vi "N-Double FFT Mesurament (Control - Init Wave&Window - Snapshot - DoubleFFT - Latency - Low Freq) RT Test.vi"() -> ()   [LabVIEW 2014]
uses:
  <vilib>/FPGAPlugInAG/sbRIO-9636/niLvFpga_Open_sbRIO-9636.vi
  <vilib>/rvi/interface/common/dynamic/niFpgaDynamicAddResources.vi
  <vilib>/Utility/error.llb/Error Cluster From Error Code.vi
  <vilib>/rvi/errors/niLvFpgaAdjustHostInterfaceError.vi
  <vilib>/rvi/interface/common/niFpgaWaitOnOcc.vi
  <vilib>/FPGAPlugInAG/Dynamic/niLvFpga_Run_Dynamic.vi
  <vilib>/FPGAPlugInAG/Dynamic/niLvFpga_Abort_Dynamic.vi
  <vilib>/FPGAPlugInAG/Dynamic/niLvFpga_Reset_Dynamic.vi
  <vilib>/FPGAPlugInAG/Dynamic/niLvFpga_Close_Dynamic.vi
  <vilib>/rvi/interface/nirviOpenFPGA/nirviOpenFPGA.xnode
  FPGA Bitfiles/LaserDistanceSen_FPGATarget_DoubleFFTMesuram_rbFcbbMisXs.lvbitx
  FPGA Target/Test VIs/Double FFT Mesurament (Control - Init Wave&Window - Snapshot - DoubleFFT - Latency - Low Freq - PARAM LEO) test.vi
  <vilib>/rvi/interface/nirviReadWriteControl/nirviReadWriteControl.xnode
  <vilib>/rvi/interface/nirviMethod/nirviMethod.xnode
  <vilib>/rvi/interface/nirviCloseFPGA/nirviCloseFPGA.xnode
  <vilib>/FPGAPlugInAG/Dynamic/niLvFpga_ConfigureFifo_Dynamic.vi
  <vilib>/rvi/errors/niLvFpgaMergeErrorWithErrorCode.vi
  <vilib>/FPGAPlugInAG/Dynamic/niLvFpga_StartFifo_Dynamic.vi
  <vilib>/rvi/interface/Simulation/niFpgaSimulationCallBeginRW.vi
  <vilib>/FPGAPlugInAG/Dynamic/niLvFpga_ReadFifo_Dynamic.vi
  NiFpgaLv.dll
panel:
  out "error out":errorcluster
  out "N-FFT":dbl[](graph)
  out "Write memory complete":bool
  in  "#Signals":u32=1
  in  "stop":bool
  in  "Initial Latency points":u32(slide)=10 scale=0.0..1249.0
  out "Elements Remaining FFT":u32
  out "Elements Remaining Signal":u32
  out "N-Signals":dbl[](graph)
  in  "Snapshot":bool
  in  "Windowing":T1(ring)
  in  "first bin":i32=15
  in  "last bin":i32=255
  in  "lower limit 2":u32(slide)=725 scale=625.0..738.0
  in  "lower limit 1":u32(slide)=100 scale=0.0..113.0
  # "WARNING:\nOnce pressed wait untill the end of operation"
  # "OFFLINE parameters"
  # "Max Detection FFT bin range"
  # "TEST"
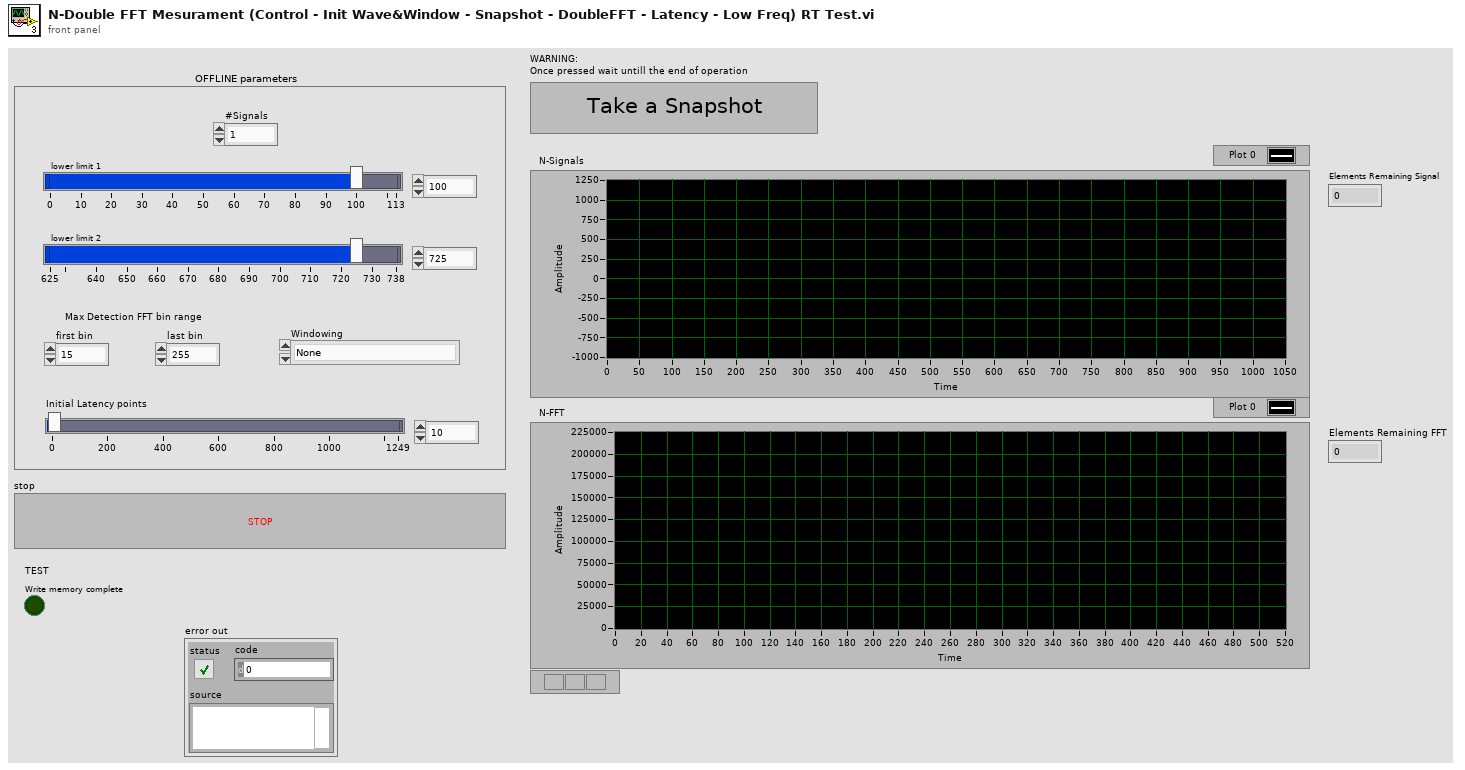
[diagram p1: front panel]
types:
  T1 = enum16{"None", "Hanning", "Hamming", "Blackman", "Blackman-Harris"}
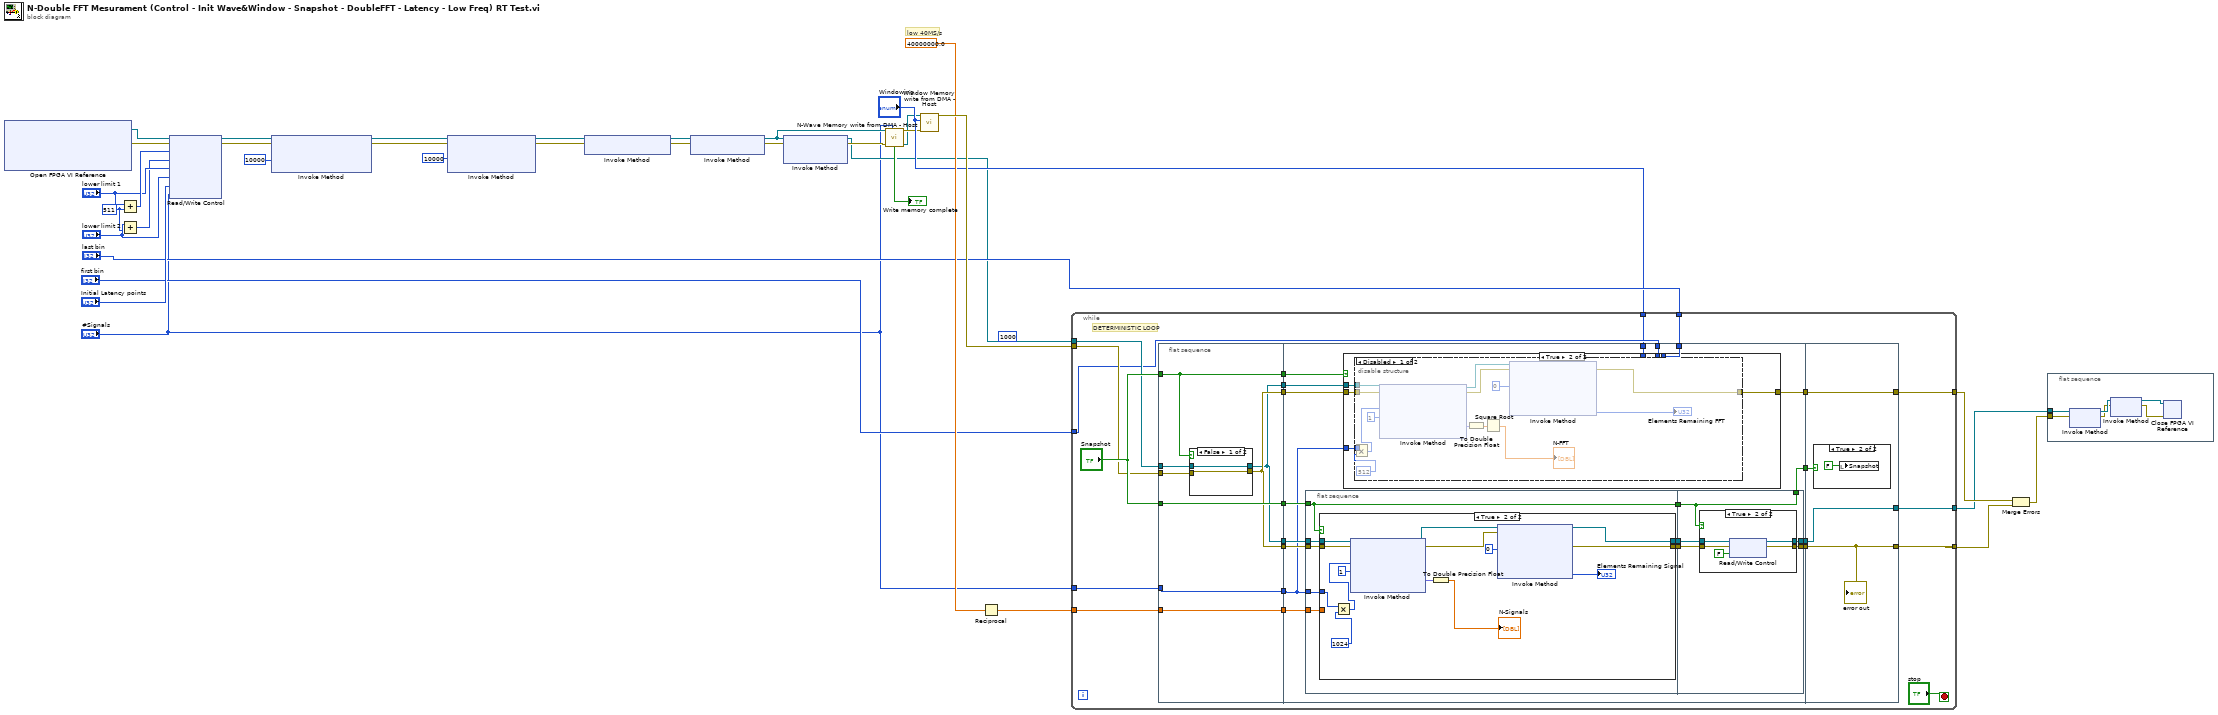
[diagram p0: block diagram]
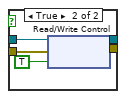
[diagram p2: hidden frame]
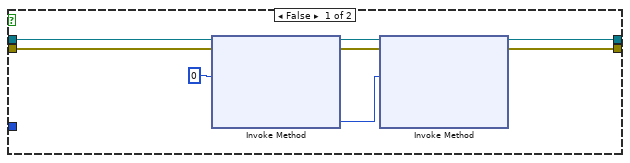
[diagram p3: hidden frame]
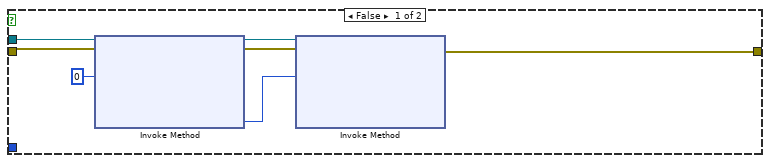
[diagram p5: hidden frame]
diagram:
  (unwired) i64 1000 ("Period")
  w32 = u32 511 ("y")
  # "low 40MS/s"
  n1 = xnode "Open FPGA VI Reference"() -> ("FPGA VI Reference Out"=w31:refnum<k20>, "error out"=w30:errorcluster)  [unwired: 2 in]
  n2 = Add(x="lower limit 1", y=w32) -> (x+y=w36:u32)
  n3 = Add(x="lower limit 2", y=w32) -> (x+y=w34:u32)
  n4 = xnode "Read/Write Control"("FPGA VI Reference In"=w31, "error in"=w30, "upper limit 1"=w36, "upper limit 2"=w34, "lower limit 1"="lower limit 1", "lower limit 2"="lower limit 2", "Latency points"="Initial Latency points", "n"="#Signals") -> ("FPGA VI Reference Out"=w28:refnum<k20>, "error out"=w27:errorcluster)
  n5 = xnode "Invoke Method"("FPGA VI Reference In"=w28, "error in"=w27, "Requested Depth"=u32 10000) -> ("FPGA VI Reference Out"=w11:refnum<k20>, "error out"=w12:errorcluster)  [unwired: 1 out]
  n6 = xnode "Invoke Method"("FPGA VI Reference In"=w11, "error in"=w12, "Requested Depth"=u32 10000) -> ("FPGA VI Reference Out"=w20:refnum<k20>, "error out"=w21:errorcluster)  [unwired: 1 out]
  n7 = xnode "Invoke Method"("FPGA VI Reference In"=w20, "error in"=w21) -> ("FPGA VI Reference Out"=w9:refnum<k20>, "error out"=w10:errorcluster)
  n8 = xnode "Invoke Method"("FPGA VI Reference In"=w9, "error in"=w10) -> ("FPGA VI Reference Out"=w2:refnum<k20>, "error out"=w19:errorcluster)
  n9 = xnode "Invoke Method"("FPGA VI Reference In"=w2, "error in"=w19) -> ("FPGA VI Reference Out"=w3:refnum<k20>, "error out"=w7:errorcluster)  [unwired: 1 in]
  n10 = call "N-Wave Memory write from DMA - Host.vi"("n"="#Signals", "error in"=w7, "FPGA VI Reference In"=w2) -> ("FPGA VI Reference Out"=w5:refnum<k20>, "error out"=w6:errorcluster, "Write memory complete"=→"Write memory complete":bool)  [unwired: 6 in]
  n11 = call "Window Memory write from DMA - Host.vi"("error in"=w6, "Enum"="Windowing", "FPGA VI Reference In"=w5) -> ("error out"=w29:errorcluster)  [unwired: 5 in, 3 out]
  n12 = Reciprocal(x=40000000.0 ("Sample Rate (S/s)")) -> (1/x=w23:dbl)
  n13 = while {
    tunnel: w3 -> [w55]
    tunnel: w29 -> [w56]
    tunnel: [w58] -> w18
    tunnel: w23 -> [w60]
    tunnel: [w59] -> w17
    tunnel: "first bin" -> [w44]
    tunnel: "last bin" -> [w43]
    tunnel: [w41] -> w13
    tunnel: "Windowing" -> [w39]
    tunnel: "#Signals" -> [w37]
    stop <- "stop" stop-if-true
    # "DETERMINISTIC LOOP"
    n14 = flat-sequence {
      tunnel: w55 -> [w64]
      tunnel: w56 -> [w65]
      tunnel: "Snapshot" -> [w62]
      tunnel: "Snapshot" -> [w67]
      tunnel: w60 -> [w68]
      tunnel: [w66] -> w54
      tunnel: [w68] -> w53
      tunnel: [w67] -> w52
      tunnel: [w62] -> w51
      tunnel: [w66] -> w50
      tunnel: [w63] -> w49
      tunnel: [w63] -> w48
      tunnel: [w61] -> w38
      tunnel: w37 -> [w61]
      tunnel: w54 -> [w89]
      tunnel: w53 -> [w88]
      tunnel: w52 -> [w82]
      tunnel: w51 -> [w85]
      tunnel: w50 -> [w84]
      tunnel: w49 -> [w83]
      tunnel: w48 -> [w90]
      tunnel: [w87] -> w47
      tunnel: [w86] -> w46
      tunnel: [w81] -> w45
      tunnel: w44 -> [w80]
      tunnel: w43 -> [w79]
      tunnel: [w78] -> w40
      tunnel: w39 -> [w77]
      tunnel: w38 -> [w76]
      tunnel: [w162] -> w58
      tunnel: [w163] -> w59
      tunnel: w47 -> [w163]
      tunnel: w46 -> [w162]
      tunnel: w45 -> [w161]
      tunnel: [w160] -> w41
      tunnel: w40 -> [w160]
      frame #0 {
        n15 = case shown="False" w62 {
          tunnel: [w69 w74] -> w66
          tunnel: w65 -> [w69 w73]
          tunnel: w64 -> [w70 w72]
          tunnel: [w70 w71] -> w63
          frame False {
          }
          frame True {
            n16 = xnode "Read/Write Control"("FPGA VI Reference In"=w72, "error in"=w73, "snapshot"=TRUE) -> ("FPGA VI Reference Out"=w71:refnum<k20>, "error out"=w74:errorcluster)
          }
        }
      }
      frame #1 {
        n17 = flat-sequence {
          tunnel: w90 -> [w100]
          tunnel: w89 -> [w99]
          tunnel: w88 -> [w98]
          tunnel: w82 -> [w95]
          tunnel: [w97] -> w93
          tunnel: [w96] -> w92
          tunnel: [w95] -> w91
          tunnel: w76 -> [w94]
          tunnel: [w125] -> w86
          tunnel: w93 -> [w127]
          tunnel: w92 -> [w126]
          tunnel: w91 -> [w124]
          tunnel: [w124] -> w81
          tunnel: [w123] -> w78
          frame #0 {
            n18 = case shown="True" w95 {
              tunnel: w100 -> [w107 w122]
              tunnel: w99 -> [w105 w121]
              tunnel: [w104 w116] -> w96
              tunnel: w98 -> [_ _]
              tunnel: [w101 w115] -> w97
              tunnel: w94 -> [_ w112]
              frame False {
                n19 = xnode "Invoke Method"("FPGA VI Reference In"=w107, "error in"=w105, "Number of Elements"=u32 0) -> ("FPGA VI Reference Out"=w103:refnum<k20>, "error out"=w102:errorcluster, "Elements Remaining"=w106:u32)  [unwired: 1 in, 1 out]
                n20 = xnode "Invoke Method"("FPGA VI Reference In"=w103, "error in"=w102, "Number of Elements"=w106) -> ("FPGA VI Reference Out"=w101:refnum<k20>, "error out"=w104:errorcluster)  [unwired: 1 in, 2 out]
              }
              frame True {
                n21 = Multiply(x=w112, y=u32 1024 ("Number of Elements")) -> (x*y=w113:u32)
                n22 = xnode "Invoke Method"("FPGA VI Reference In"=w122, "error in"=w121, "Number of Elements"=w113, "Timeout (ms)"=1) -> ("FPGA VI Reference Out"=w118:refnum<k20>, "error out"=w117:errorcluster, "Data"=w120:fxp<+/-,12,12>[])  [unwired: 1 out]
                n23 = To Double Precision Float(number=w120) -> (double precision float=→"N-Signals":dbl[])
                n24 = xnode "Invoke Method"("FPGA VI Reference In"=w118, "error in"=w117, "Number of Elements"=u32 0) -> ("FPGA VI Reference Out"=w115:refnum<k20>, "error out"=w116:errorcluster, "Elements Remaining"=→"Elements Remaining Signal":u32)  [unwired: 1 in, 1 out]
              }
            }
          }
          frame #1 {
            n25 = case shown="True" w124 {
              tunnel: [w129 w132] -> w125
              tunnel: w127 -> [w128 w133]
              tunnel: w126 -> [w129 w131]
              tunnel: [w128 w130] -> w123
              frame False {
              }
              frame True {
                n26 = xnode "Read/Write Control"("FPGA VI Reference In"=w133, "error in"=w131, "snapshot"=FALSE) -> ("FPGA VI Reference Out"=w130:refnum<k20>, "error out"=w132:errorcluster)
              }
            }
          }
        }
        n27 = case shown="True" w85 {
          tunnel: w83 -> [w140 w144]
          tunnel: w84 -> [w137 w145]
          tunnel: [w136 w143] -> w87
          tunnel: w80 -> [_ _]
          tunnel: w79 -> [_ _]
          tunnel: w77 -> [_ _]
          tunnel: w76 -> [_ w142]
          frame False {
            n28 = xnode "Invoke Method"("FPGA VI Reference In"=w140, "error in"=w137, "Number of Elements"=u32 0) -> ("FPGA VI Reference Out"=w138:refnum<k20>, "error out"=w135:errorcluster, "Elements Remaining"=w139:u32)  [unwired: 1 in, 1 out]
            n29 = xnode "Invoke Method"("FPGA VI Reference In"=w138, "error in"=w135, "Number of Elements"=w139) -> ("error out"=w136:errorcluster)  [unwired: 1 in, 3 out]
          }
          frame True {
            n30 = disable-structure shown="Disabled" {
              disable-tunnel: w145 -> [w157 _]
              disable-tunnel: w144 -> [w156 _]
              disable-tunnel: [w155 _] -> w143
              disable-tunnel: w142 -> [w148 _]
              frame Disabled {
                n31 = Multiply(x=w148, y=u32 512 ("Number of Elements")) -> (x*y=w149:u32)
                n32 = xnode "Invoke Method"("FPGA VI Reference In"=w156, "error in"=w157, "Number of Elements"=w149, "Timeout (ms)"=1) -> ("FPGA VI Reference Out"=w153:refnum<k20>, "error out"=w154:errorcluster, "Data"=w159:fxp<+,44,44>[])  [unwired: 1 out]
                n33 = To Double Precision Float(number=w159) -> (double precision float=w158:dbl[])
                n34 = Square Root(x=w158) -> (sqrt(x)=→"N-FFT":dbl[])
                n35 = xnode "Invoke Method"("FPGA VI Reference In"=w153, "error in"=w154, "Number of Elements"=u32 0) -> ("error out"=w155:errorcluster, "Elements Remaining"=→"Elements Remaining FFT":u32)  [unwired: 1 in, 2 out]
              }
              frame Enabled {
              }
            }
          }
        }
      }
      frame #2 {
        n36 = case shown="True" w161 {
          frame False {
          }
          frame True {
            n37 = local write "Snapshot"(FALSE ("Snapshot")) -> ()
          }
        }
        "error out" <- w162
      }
    }
  }
  n38 = Merge Errors(w17, w18) -> (w24:errorcluster)
  n39 = flat-sequence {
    tunnel: w24 -> [w170]
    tunnel: w13 -> [w165]
    frame #0 {
      n40 = xnode "Invoke Method"("FPGA VI Reference In"=w165, "error in"=w170) -> ("FPGA VI Reference Out"=w167:refnum<k20>, "error out"=w166:errorcluster)
      n41 = xnode "Invoke Method"("FPGA VI Reference In"=w167, "error in"=w166) -> ("FPGA VI Reference Out"=w168:refnum<k20>, "error out"=w169:errorcluster)
      n42 = xnode "Close FPGA VI Reference"("FPGA VI Reference In"=w168, "error in"=w169) -> ()  [unwired: 1 out]
    }
  }
